vi "StringArray.vi"(7 "Array Name":string, 8 "Input":string[](array[string]), 11 "Carry":string) -> (3 "Output":string)   [LabVIEW 2016]
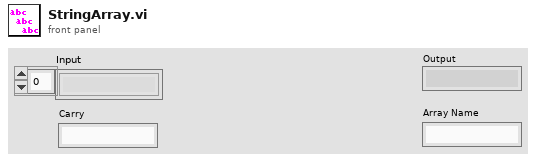
[diagram p1: front panel]
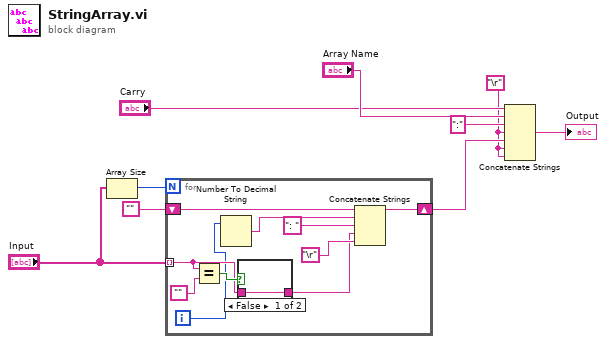
[diagram p0: block diagram]
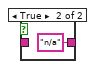
[diagram p2: hidden frame]
diagram:
  w1 = "\r"
  n1 = Array Size(array="Input") -> (size(s)=w8:i32)
  n2 = for {
    N: w8 -> [_]
    tunnel: "Input" -> [w11] mode=indexing
    shift-right: [w16] -> w2
    shift-left: "" -> [w15]
    i -> [w10]
    n3 = Equal?(x=w11, y="") -> (x = y?=w13:bool)
    n4 = Number To Decimal String(number=w10) -> (decimal integer string=w19:string)  [unwired: 1 in]
    n5 = case shown="False" w13 {
      tunnel: [w20 "n/a"] -> w12
      tunnel: w11 -> [w20 _]
      frame False {
      }
      frame True {
      }
    }
    n6 = Concatenate Strings(w15, w19, ": " ("string"), w12, "\r") -> (w16:string)
  }
  n7 = Concatenate Strings("Carry", "Array Name", ":" ("string"), w1, w2, w1, w1) -> (→"Output":string)
